vi "Convert to Base64.vi"(3 "String":string) -> (1 "Base64 String":string)   [LabVIEW 2015, in "Front Panel Publisher.lvlib"]
doc: "This VI converts a string to its Base64 equivalent. Base64 strings are commonly used in Internet protocols such as HTTP, SMTP, etc."
uses:
  Front Panel Publisher.lvlib
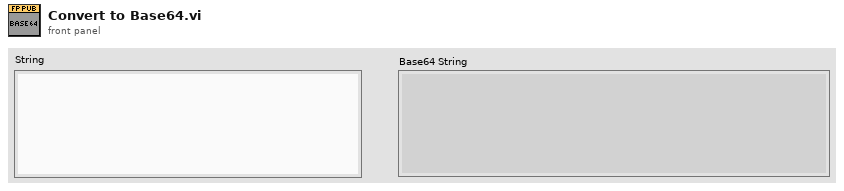
[diagram p1: front panel]
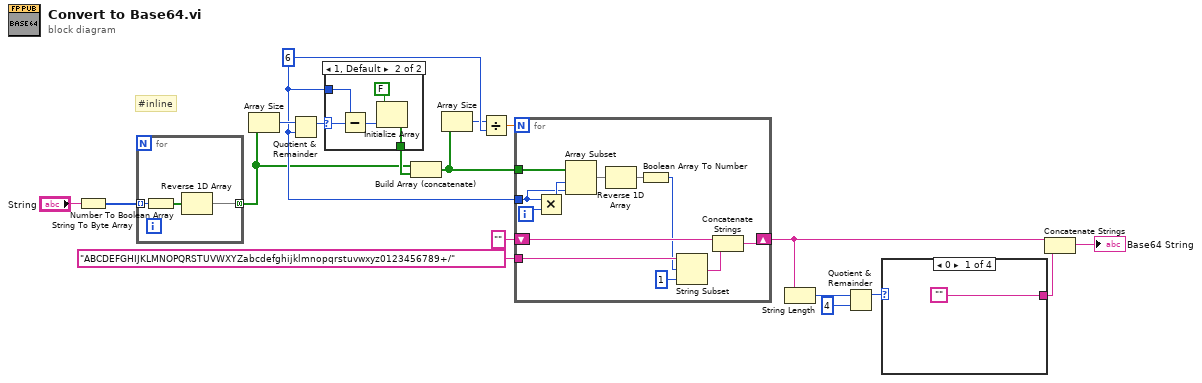
[diagram p0: block diagram]
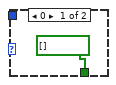
[diagram p2: hidden frame]
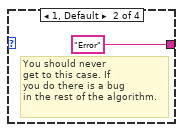
[diagram p3: hidden frame]
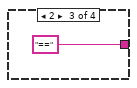
[diagram p4: hidden frame]
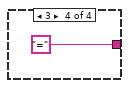
[diagram p5: hidden frame]
diagram:
  w4 = 6 ("y")
  # "#inline"
  n1 = String To Byte Array(string="String") -> (unsigned byte array=w17:u8[])
  n2 = for {
    tunnel: w17 -> [w21] mode=indexing
    tunnel: [w19] -> w1 mode=concatenating
    n3 = Number To Boolean Array(number=w21) -> (Boolean array=w20:bool[])
    n4 = Reverse 1D Array(array=w20) -> (reversed array=w19:bool[])
  }
  n5 = Array Size(array=w1) -> (size(s)=w7:i32)
  n6 = Quotient & Remainder(x=w7, y=w4) -> (x-y*floor(x/y)=w6:i32)  [unwired: 1 out]
  n7 = case shown="1, Default" w6 {
    selector: w6 -> [_ w26]
    tunnel: [bool[] [] w23] -> w5
    tunnel: w4 -> [_ w25]
    frame 0 {
    }
    frame 1, Default {
      n8 = Subtract(x=w25, y=w26) -> (x-y=w27:i32)
      n9 = Initialize Array(FALSE, w27) -> (w23:bool[])
    }
  }
  n10 = Build Array (concatenate)(w1, w5) -> (w3:bool[])
  n11 = Array Size(array=w3) -> (size(s)=w2:i32)
  n12 = Divide(x=w2, y=w4) -> (x/y=w8:dbl)
  n13 = for {
    N: w8 -> [_]
    tunnel: w3 -> [w38]
    tunnel: w4 -> [w36]
    tunnel: "ABCDEFGHIJKLMNOPQRSTUVWXYZabcdefghijklmnopqrstuvwxyz0123456789+/" -> [w35]
    shift-right: [w33] -> w10
    shift-left: "" -> [w32]
    i -> [w39]
    n14 = Multiply(x=w36, y=w39) -> (x*y=w37:i32)
    n15 = Array Subset(array=w38, index=w37, length=w36) -> (w28:bool[])
    n16 = Reverse 1D Array(array=w28) -> (reversed array=w29:bool[])
    n17 = Boolean Array To Number(Boolean array=w29) -> (number=w30:u32)
    n18 = String Subset(string=w35, offset (0)=w30, length (rest)=1 ("length (rest)")) -> (substring=w31:string)
    n19 = Concatenate Strings(w32, w31) -> (w33:string)
  }
  n20 = String Length(string=w10) -> (length=w14:i32)
  n21 = Quotient & Remainder(x=w14, y=4) -> (x-y*floor(x/y)=w12:i32)  [unwired: 1 out]
  n22 = case shown="0" w12 {
    tunnel: ["" "Error" "==" "="] -> w11
    frame 0 {
    }
    frame 1, Default {
      # "You should never\nget to this case. If\nyou do there is a bug\nin the rest of the algorithm."
    }
    frame 2 {
    }
    frame 3 {
    }
  }
  n23 = Concatenate Strings(w10, w11) -> (→"Base64 String":string)
